vi "Actor Core.vi"(8 "error in":errorcluster, 11 "Host MSS Test Actor in":refnum<class "Host MSS Test Actor.lvclass">) -> (0 "error out":errorcluster, 3 "Actor out":refnum<class "Actor.lvclass">)   [LabVIEW 2023, in "Host MSS Test Actor.lvlib" / "Host MSS Test Actor.lvclass"]
doc: "(<B>Filename</B>: Actor Framework.lvlib:Actor.lvclass:Actor Core.vi)\n\nReceives messages to the actor, reacts to them, and initiates any error handling that may shut the actor down.\n\nDescendant classes may override this VI to append parallel tasks for the actor to complete while it handles messages. Overrides use the Call Parent Class Method node."
uses:
  Host MSS Test Actor.lvclass
  <vilib>/ActorFramework/Actor/Actor.lvclass
  <vilib>/ni/Actors/Network Endpoint Actors/Notifying Nested Endpoint/Notifying Nested Endpoint.lvclass
  <vilib>/ActorFramework/Actor/Actor.lvclass/Actor.ctl
  <vilib>/ActorFramework/Message Enqueuer/Message Enqueuer.lvclass/Message Enqueuer.ctl
  Host MSS Test Actor.lvclass/Host MSS Test Actor.ctl
  <vilib>/ni/Actors/Network Endpoint Actors/Network Endpoint/Network Endpoint/Network Endpoint.lvclass/Network Endpoint.ctl
  Host MSS Test Actor Messages/Init Series Msg/Init Series Msg.lvclass/Init Series Msg.ctl
  <vilib>/ActorFramework/Message Enqueuer/Init from Existing Queue.vi
  <vilib>/ActorFramework/Message Enqueuer/Enqueue.vi
  Host MSS Test Actor Messages/Init Series Msg/Init Series Msg.lvclass
  Host MSS Test Actor Messages/Start Series Msg/Start Series Msg.lvclass
  <vilib>/ActorFramework/Stop Msg/Stop Msg.lvclass
  <vilib>/Utility/LVClass/Get LV Class Name.vi
  <resource>/AFDebug/Generate Trace for Message.vi
  <vilib>/ActorFramework/Message Priority Queue/Priority Enqueue.vi
  <vilib>/ActorFramework/Message Enqueuer/Message Enqueuer.lvclass
  <vilib>/ni/Actors/Network Endpoint Actors/Network Endpoint/Network Endpoint/Network Endpoint.lvclass
panel:
  in  "Stop Button":bool
  in  "Start Series Button":bool
  in  "Init Series Button":bool
  in  "Kill CRIO Button":bool
  out "Connected":bool
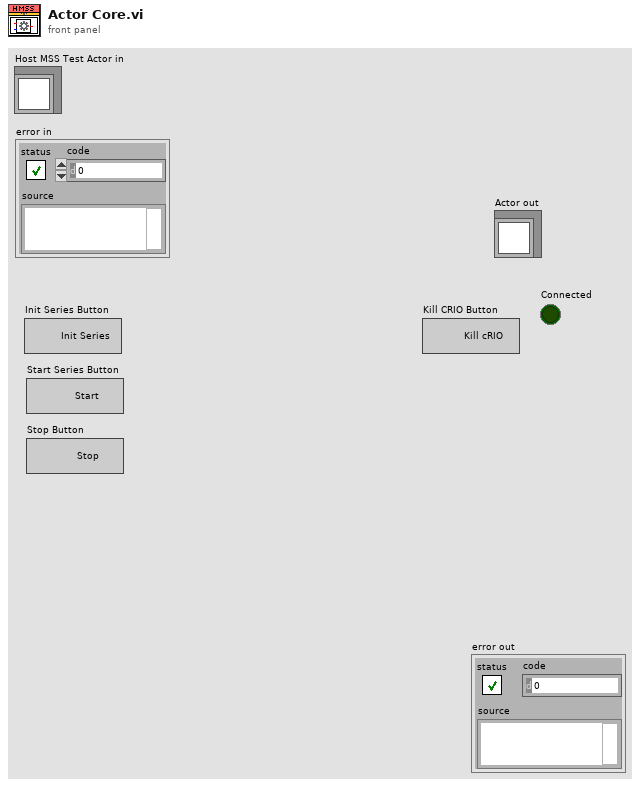
[diagram p1: front panel]
types:
  T1 = cluster{"Stop":refnum<user-event>, "Connected":refnum<user-event>}
  T2 = map{string, refnum<class "Message Enqueuer.lvclass">}
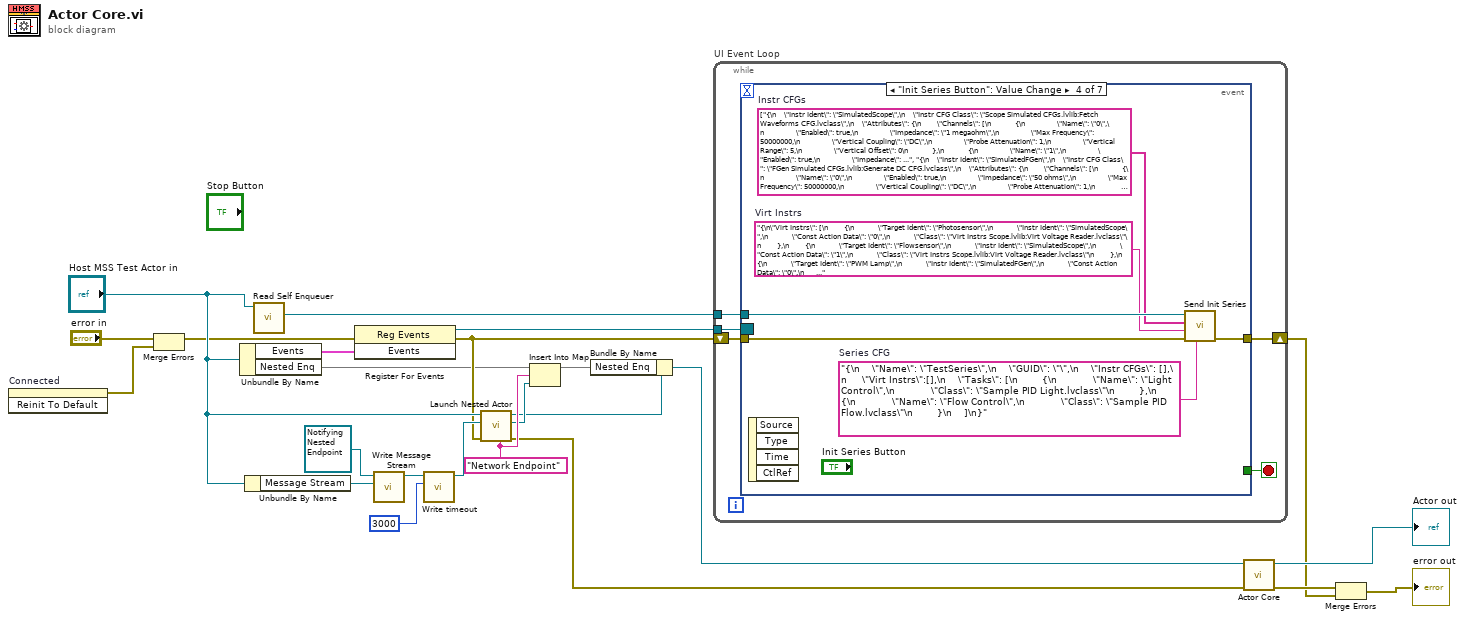
[diagram p0: block diagram]
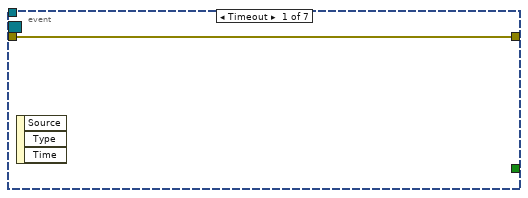
[diagram p2: hidden frame]
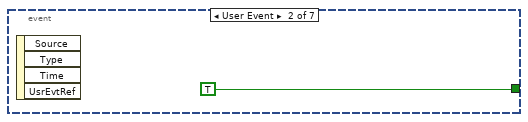
[diagram p3: hidden frame]
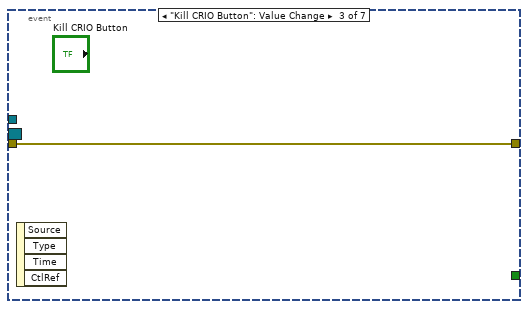
[diagram p4: hidden frame]
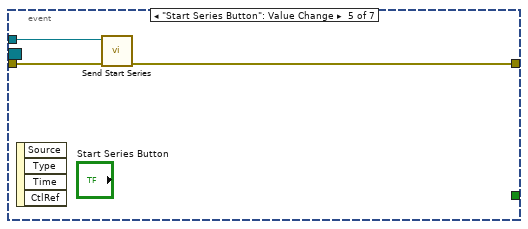
[diagram p5: hidden frame]
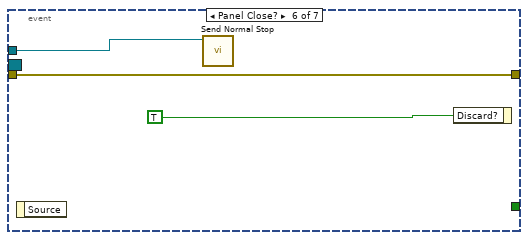
[diagram p6: hidden frame]
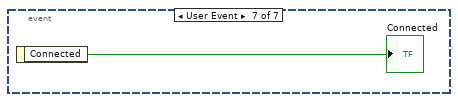
[diagram p7: hidden frame]
diagram:
  w11 = "Network Endpoint" ("Debug Alias")
  n1 = invoke on="Connected" class="Bool (strict)" method="Reinit To Default"() -> (error out=w1:errorcluster)  [unwired: 3 in, 2 out]
  n2 = Merge Errors("error in", w1) -> (w2:errorcluster)
  n3 = Unbundle By Name("Host MSS Test Actor in") -> ("Events"=w22:T1, "Nested Enq"=w3:T2)
  n4 = Unbundle By Name("Host MSS Test Actor in") -> ("Message Stream"=w15:refnum<class "Message Stream.lvclass">)
  n5 = call <vilib>:"Read Self Enqueuer.vi"("Actor"="Host MSS Test Actor in") -> ("Self Enqueuer"=w14:refnum<class "Message Enqueuer.lvclass">)  [unwired: 10 in]
  n6 = register-events(error in=w2, w22) -> (reference out=w21:refnum<event-registration>, error out=w7:errorcluster)  [unwired: 1 in]
  n7 = call <vilib>:"Write Message Stream.vi"("Message Stream"=w15, "Network Endpoint in"=refnum<class "Notifying Nested Endpoint.lvclass"> refnum ("Notifying Nested Endpoint.lvclass")) -> ("Network Endpoint out"=w17:refnum<class "Notifying Nested Endpoint.lvclass">)  [unwired: 9 in]
  n8 = call <vilib>:"Write timeout.vi"("timeout"=3000, "Network Endpoint in"=w17) -> ("Network Endpoint out"=w13:refnum<class "Notifying Nested Endpoint.lvclass">)  [unwired: 9 in]
  n9 = call <vilib>:"Launch Nested Actor.vi"("Debug Alias"=w11, "error in (no error)"=w7, "Nested Actor"=w13, "Caller Actor in"="Host MSS Test Actor in") -> ("error out"=w6:errorcluster, "Nested Actor's Enqueuer"=w10:refnum<class "Message Enqueuer.lvclass">, "Caller Actor out"=w9:refnum<class "Host MSS Test Actor.lvclass">)  [unwired: 5 in]
  n10 = Insert Into Map(map in=w3, key=w11, value=w10) -> (map out=w4:T2)  [unwired: 2 out]
  n11 = Bundle By Name(cluster=w9, "Nested Enq"=w4) -> (w5:refnum<class "Host MSS Test Actor.lvclass">)
  n12 = while "UI Event Loop" {
    tunnel: w21 -> [w29]
    shift-right: [w27] -> w19
    shift-left: w7 -> [w28]
    tunnel: w14 -> [w25]
    stop <- w26 stop-if-true
    n13 = event shown="[3] \"Init Series Button\": Value Change" {
      selector: w29 -> [_ _ _ _ _ _ _]
      dyn-events: _ -> [_ _ _ _ _ _ _]
      timeout: _ -> [_ _ _ _ _ _ _]
      tunnel: w28 -> [w30 _ w32 w38 w40 w42 _]
      tunnel: [w30 _ w32 w37 w39 w42 _] -> w27
      tunnel: [_ TRUE _ _ _ _ _] -> w26
      tunnel: w25 -> [_ _ _ w36 w41 w43 _]
      event Timeout {
        n14 = event-data() -> ()  [unwired: 1 in, 3 out]
      }
      event User Event {
        n15 = event-data() -> ()  [unwired: 1 in, 4 out]
      }
      event "Kill CRIO Button": Value Change {
        n16 = event-data() -> ()  [unwired: 1 in, 4 out]
      }
      event "Init Series Button": Value Change {
        w34 = "{\n\"Virt Instrs\": [\n        {\n            \"Target Ident\": \"Photosensor\",\n            \"Instr Ident\": \"SimulatedScope\",\n            \"Const Action Data\": \"0\",\n            \"Class\": \"Virt Instrs Scope.lvlib:Virt Voltage Reader.lvclass\"\n        },\n        {\n            \"Target Ident\": \"Flowsensor\",\n            \"Instr Ident\": \"SimulatedScope\",\n            \"Const Action Data\": \"1\",\n            \"Class\": \"Virt Instrs Scope.lvlib:Virt Voltage Reader.lvclass\"\n        },\n        {\n            \"Target Ident\": \"PWM Lamp\",\n            \"Instr Ident\": \"SimulatedFGen\",\n            \"Const Action Data\": \"0\",\n            \"Class\": \"Virt Instrs FGen.lvlib:Virt Voltage Generator.lvclass\"\n        },\n        {\n            \"Target Ident\": \"PWM Flow\",\n            \"Instr Ident\": \"Sim9472\",\n            \"Const Action Data\": \"0\",\n            \"Class\": \"Virt Instrs DIO.lvlib:Virt DAQmx Fixed Freq PWM Generator.lvclass\"\n        }\n    ]\n}"  # Virt Instrs
        w33 = string[] ["{\n    \"Instr Ident\": \"SimulatedScope\",\n    \"Instr CFG Class\": \"Scope Simulated CFGs.lvlib:Fetch Waveforms CFG.lvclass\",\n    \"Attributes\": {\n        \"Channels\": [\n            {\n                \"Name\": \"0\",\n                \"Enabled\": true,\n                \"Impedance\": \"1 megaohm\",\n                \"Max Frequency\": 50000000,\n                \"Vertical Coupling\": \"DC\",\n                \"Probe Attenuation\": 1,\n                \"Vertical Range\": 5,\n                \"Vertical Offset\": 0\n            },\n            {\n                \"Name\": \"1\",\n                \"Enabled\": true,\n                \"Impedance\": \"50 ohms\",\n                \"Max Frequency\": 50000000,\n                \"Vertical Coupling\": \"DC\",\n                \"Probe Attenuation\": 1,\n                \"Vertical Range\": 5,\n                \"Vertical Offset\": 0\n            },\n            {\n                \"Name\": \"2\",\n                \"Enabled\": false,\n                \"Impedance\": \"50 ohms\",\n                \"Max Frequency\": 50000000,\n                \"Vertical Coupling\": \"DC\",\n                \"Probe Attenuation\": 1,\n                \"Vertical Range\": 5,\n                \"Vertical Offset\": 0\n            },\n            {\n                \"Name\": \"3\",\n                \"Enabled\": false,\n                \"Impedance\": \"50 ohms\",\n                \"Max Frequency\": 50000000,\n                \"Vertical Coupling\": \"DC\",\n                \"Probe Attenuation\": 1,\n                \"Vertical Range\": 1.4,\n                \"Vertical Offset\": 0\n            },\n            {\n                \"Name\": \"4\",\n                \"Enabled\": false,\n                \"Impedance\": \"50 ohms\",\n                \"Max Frequency\": 50000000,\n                \"Vertical Coupling\": \"DC\",\n                \"Probe Attenuation\": 1,\n                \"Vertical Range\": 5,\n                \"Vertical Offset\": 0\n            },\n            {\n                \"Name\": \"5\",\n                \"Enabled\": false,\n                \"Impedance\": \"50 ohms\",\n                \"Max Frequency\": 50000000,\n                \"Vertical Coupling\": \"DC\",\n                \"Probe Attenuation\": 1,\n                \"Vertical Range\": 5,\n                \"Vertical Offset\": 0\n            },\n            {\n                \"Name\": \"6\",\n                \"Enabled\": false,\n                \"Impedance\": \"50 ohms\",\n                \"Max Frequency\": 50000000,\n                \"Vertical Coupling\": \"DC\",\n                \"Probe Attenuation\": 1,\n                \"Vertical Range\": 5,\n                \"Vertical Offset\": 0\n            },\n            {\n                \"Name\": \"7\",\n                \"Enabled\": false,\n                \"Impedance\": \"50 ohms\",\n                \"Max Frequency\": 50000000,\n                \"Vertical Coupling\": \"DC\",\n                \"Probe Attenuation\": 1,\n                \"Vertical Range\": 5,\n                \"Vertical Offset\": 0\n            }\n        ],\n        \"Horizontal\": {\n            \"Enforce Realtime\": true,\n            \"Number of Records\": 1,\n            \"Min Sample Rate\": 100000,\n            \"Reference Position\": 50,\n            \"Min Record Length\": 1000\n        },\n        \"Acquire\": {\n            \"Type\": \"Normal\",\n            \"NumSamples\": 1000,\n            \"Fetch Relative To\": \"Read Pointer\"\n        },\n        \"Export Signal\": {\n            \"Signal Identifier\": \"None\",\n            \"Signal\": \"None\",\n            \"Output Terminal\": \"None\"\n        },\n        \"Trigger\": {\n            \"Type\": \"Immediate\",\n            \"Slope\": \"Positive\",\n            \"Source\": \"RTSI 0\",\n            \"Holdoff\": 0,\n            \"Delay\": 0\n        }\n    }\n}", "{\n    \"Instr Ident\": \"SimulatedFGen\",\n    \"Instr CFG Class\": \"FGen Simulated CFGs.lvlib:Generate DC CFG.lvclass\",\n    \"Attributes\": {\n        \"Channels\": [\n            {\n                \"Name\": \"0\",\n                \"Enabled\": true,\n                \"Impedance\": \"50 ohms\",\n                \"Max Frequency\": 50000000,\n                \"Vertical Coupling\": \"DC\",\n                \"Probe Attenuation\": 1,\n                \"Vertical Range\": 10,\n                \"Vertical Offset\": 0\n            },\n            {\n                \"Name\": \"1\",\n                \"Enabled\": false,\n                \"Impedance\": \"50 ohms\",\n                \"Max Frequency\": 50000000,\n                \"Vertical Coupling\": \"DC\",\n                \"Probe Attenuation\": 1,\n                \"Vertical Range\": 0.2,\n                \"Vertical Offset\": 0\n            }\n        ],\n        \"Horizontal\": {\n            \"Enforce Realtime\": true,\n            \"Number of Records\": 1,\n            \"Min Sample Rate\": 100000,\n            \"Reference Position\": 50,\n            \"Min Record Length\": 1000\n        },\n        \"Acquire\": {\n            \"Type\": \"Normal\"\n        },\n        \"Export Signal\": {\n            \"Enabled\": false,\n            \"Signal Identifier\": \"None\",\n            \"Signal\": \"None\",\n            \"Output Terminal\": \"None\"\n        },\n        \"Trigger\": {\n            \"Type\": \"Digital\",\n            \"Source\": \"RTSI 0\",\n            \"Holdoff\": 0,\n            \"Delay\": 0\n        }\n    }\n}", "{\n    \"Instr Ident\": \"Sim9472\",\n    \"Instr CFG Class\": \"DAQmx Simulated CFGs.lvlib:DO DAQmx PWM Fixed Freq CFG.lvclass\",\n    \"Attributes\": {\n        \"Channels\": [\n            {\n                \"Name\": \"ctr0\",\n                \"Enabled\": true,\n                \"Duty Cycle\": 0.5,\n                \"Frequency\": 600,\n                \"Units\": \"Hz\",\n                \"Idle State\": \"Low\",\n                \"Initial Delay\": 0\n            },\n            {\n                \"Name\": \"ctr1\",\n                \"Enabled\": false,\n                \"Duty Cycle\": 0.5,\n                \"Frequency\": 1,\n                \"Units\": \"Hz\",\n                \"Idle State\": \"Low\",\n                \"Initial Delay\": 0\n            },\n            {\n                \"Name\": \"ctr2\",\n                \"Enabled\": false,\n                \"Duty Cycle\": 0.5,\n                \"Frequency\": 1,\n                \"Units\": \"Hz\",\n                \"Idle State\": \"Low\",\n                \"Initial Delay\": 0\n            },\n            {\n                \"Name\": \"ctr3\",\n                \"Enabled\": false,\n                \"Duty Cycle\": 0.5,\n                \"Frequency\": 1,\n                \"Units\": \"Hz\",\n                \"Idle State\": \"Low\",\n                \"Initial Delay\": 0\n            }\n        ],\n        \"Timing\": {\n            \"Samples per Channel\": 1000,\n            \"Sample Mode\": \"Continuous Samples\",\n            \"Sample Rate\": 0,\n            \"Sample Clock Source\": \"Implicit\",\n            \"Active Edge\": \"Rising\"\n        },\n        \"Trigger\": {\n            \"Trigger Type\": \"No Trigger\"\n        }\n    }\n}"]  # Instr CFGs
        w35 = "{\n    \"Name\": \"TestSeries\",\n    \"GUID\": \"\",\n    \"Instr CFGs\": [],\n     \"Virt Instrs\":[],\n    \"Tasks\": [\n        {\n            \"Name\": \"Light Control\",\n            \"Class\": \"Sample PID Light.lvclass\"\n        },\n        {\n            \"Name\": \"Flow Control\",\n            \"Class\": \"Sample PID Flow.lvclass\"\n        }\n    ]\n}"  # Series CFG
        n17 = event-data() -> ()  [unwired: 1 in, 4 out]
        n18 = call "Send Init Series.vi"("Series CFG"=w35, "error in (no error)"=w38, "Virt Instrs CFG"=w34, "Instr CFGs"=w33, "Message Enqueuer"=w36) -> ("error out"=w37:errorcluster)  [unwired: 5 in, 1 out]
      }
      event "Start Series Button": Value Change {
        n19 = event-data() -> ()  [unwired: 1 in, 4 out]
        n20 = call "Send Start Series.vi"("error in (no error)"=w40, "Message Enqueuer"=w41) -> ("error out"=w39:errorcluster)  [unwired: 8 in, 1 out]
      }
      event Panel Close? {
        n21 = event-data() -> ()  [unwired: 1 in, 1 out]
        n22 = call <vilib>:"Send Normal Stop.vi"("Message Enqueuer"=w43) -> ()  [unwired: 10 in, 1 out]
        n23 = event-data("Discard?"=TRUE) -> ()  [unwired: 1 in, 1 out]
      }
      event User Event {
        n24 = event-data() -> ("Connected"=→"Connected":bool)  [unwired: 1 in]
      }
    }
  }
  n25 = call-parent "Actor Core.vi"("error in"=w6, "Actor in"=w5) -> ("error out"=w24:errorcluster, "Actor out"=→"Actor out":refnum<class "Actor.lvclass">)  [unwired: 8 in]
  n26 = Merge Errors(w24, w19) -> (→"error out":errorcluster)
